vi "Scan Callers.vi"(8 "error in (no error)":errorcluster, 11 "WorkSpace / Repo path":path) -> (0 "error out":errorcluster)   [LabVIEW 2019, in "Hawkeye.lvlib"]
uses:
  Hawkeye.lvlib
panel:
  out "Dependency Chain [] 2":string[](array[string])
  in  "WorkSpace / Repo path 2":path
  out "Array 2":string[](array[string])
  out "Array 3":string[][](array[string])
  in  "Scan":bool
  in  "Status":string
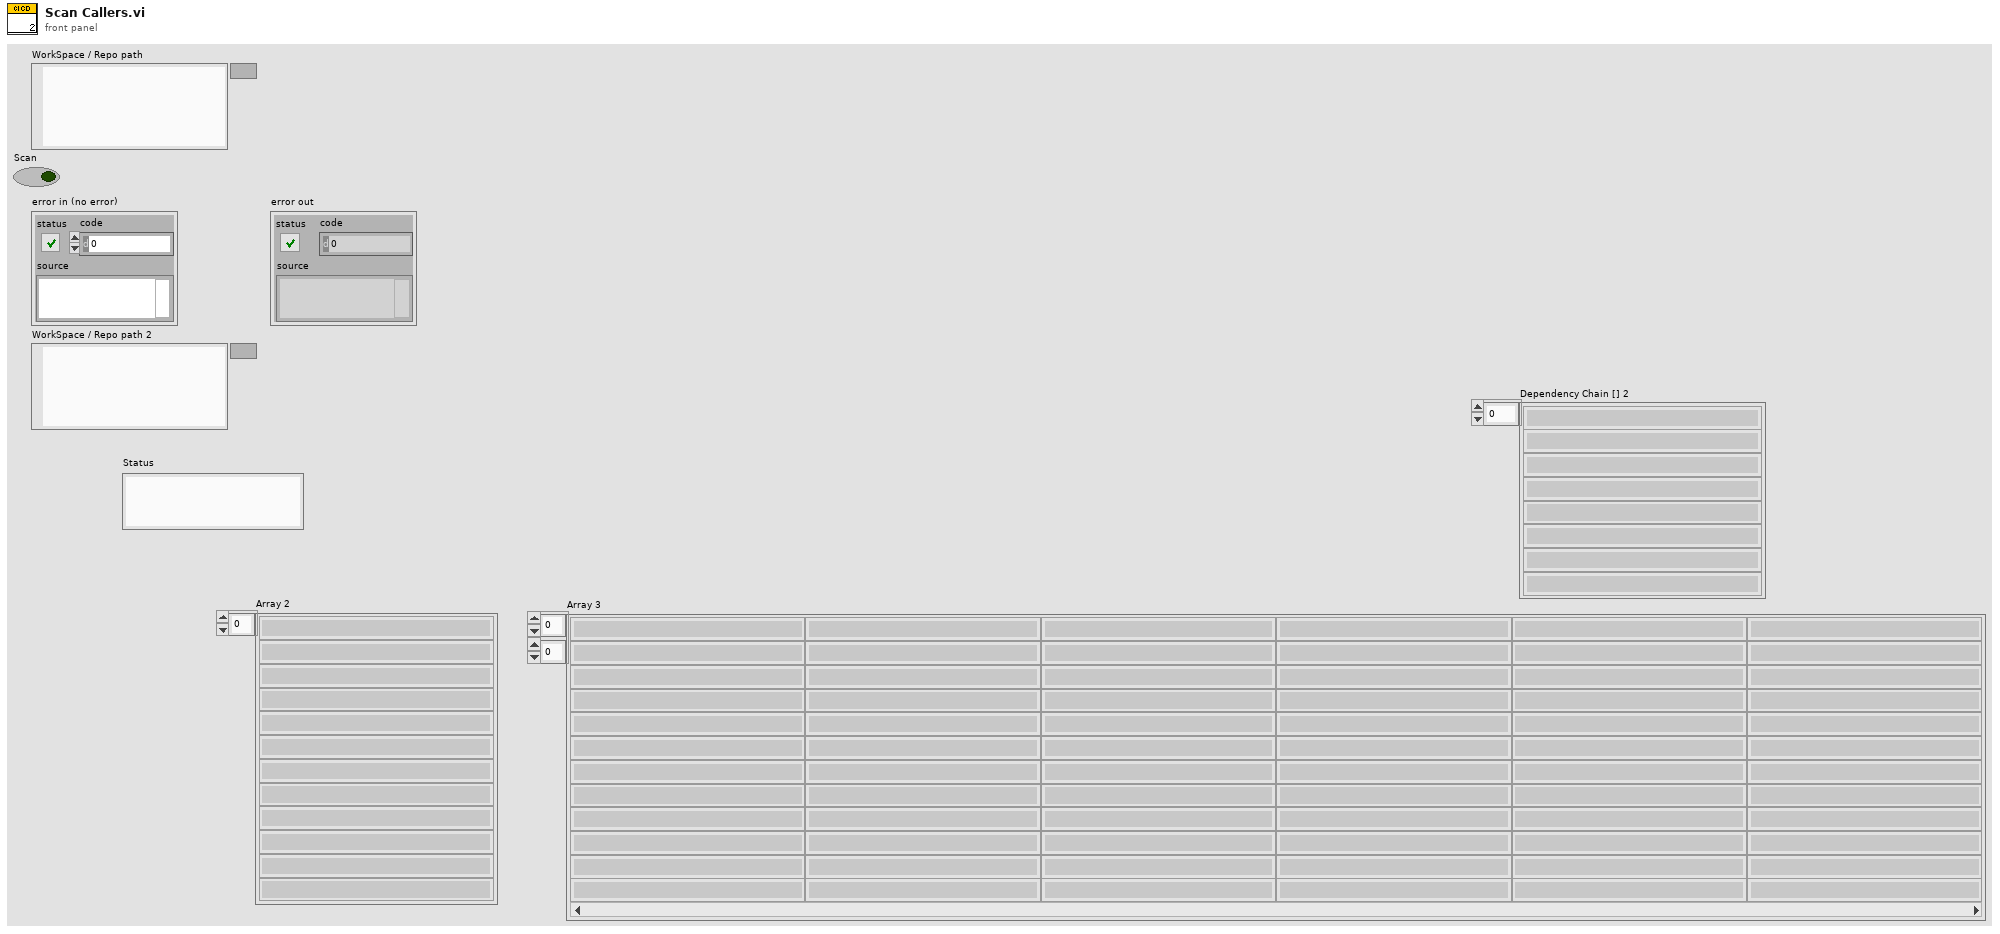
[diagram p1: front panel]
types:
  T1 = cluster{"VI Path":path, "Callees":set{string}, "LVLib/LVClass Name":string}[]
  T2 = enum16{"open", "replace", "create", "open or create", "replace or create", "replace or create with confirmation"}
  T3 = cluster{"VI Path":path, "Callees":set{string}, "LVLib/LVClass Name":string}
  T4 = typedef "NI_FileType.lvlib/LVFileType.ctl" = enum32{"Invalid file", "Unknown type", "Instrument", "Control", "Polymorphic VI", "Project", "Library", "LVClass", "XControl", "XNode", "Shared library", ".NET assembly", "ActiveX interface", "CIN", "Run-time menu", "Palette menu", "Help file", "LLB", "XNode Edit Dependency", "Class Private Data Control", "Statechart", "MathScript .m file", "Ladder Diagram", "LVLibp", "XNode Build Dependency"}
  T5 = cluster{"path":path, "delimited name":string, "type":T4, "iState":u32, "iStyle":u16, "wStyle":u16, "buttons":u16, "viflags":u32, "viflags2":u32, "links":u32[]}[]
  T6 = cluster{"path":path, "delimited name":string, "type":T4, "iState":u32, "iStyle":u16, "wStyle":u16, "buttons":u16, "viflags":u32, "viflags2":u32, "links":u32[]}
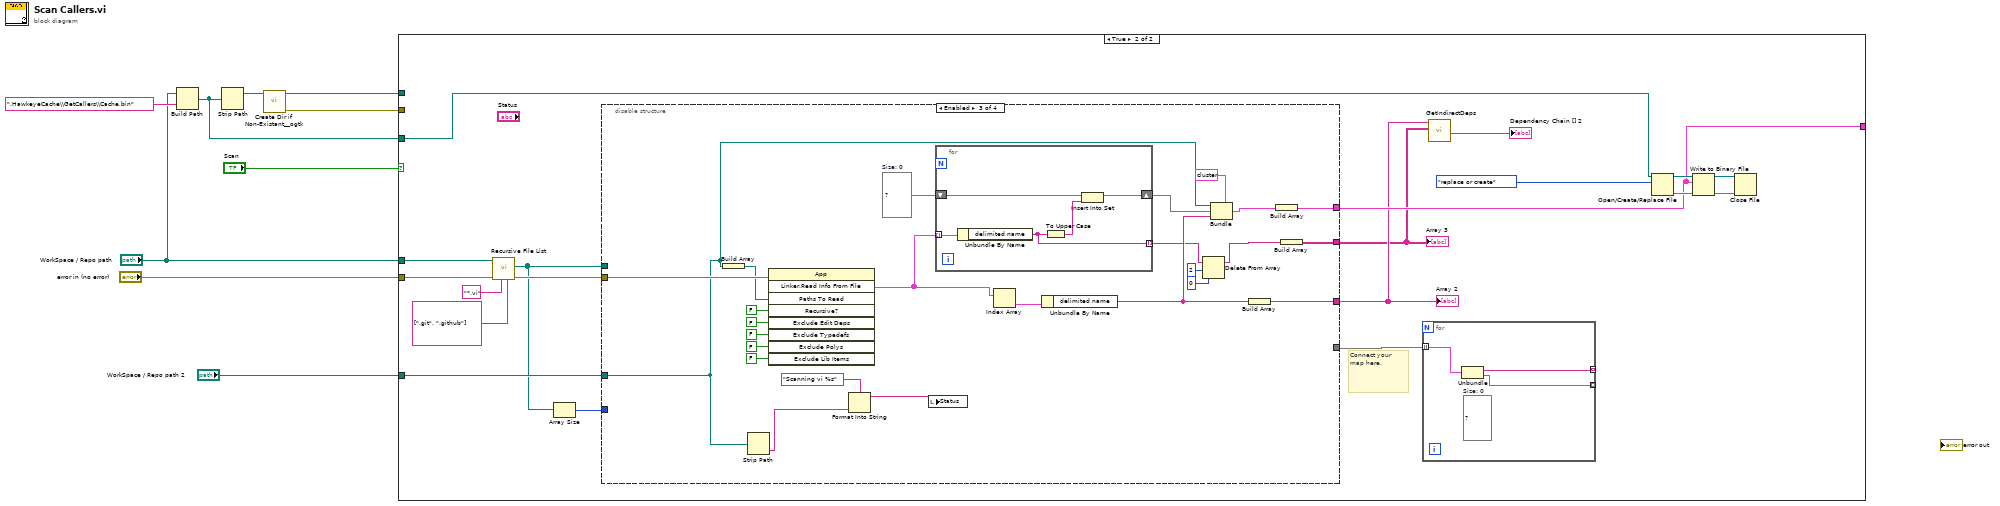
[diagram p0: block diagram]
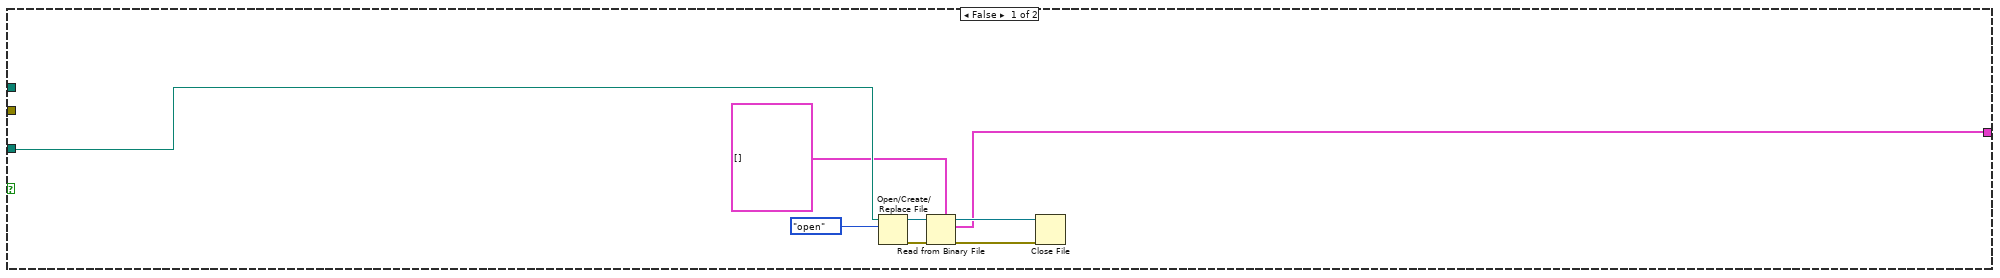
[diagram p2: hidden frame]
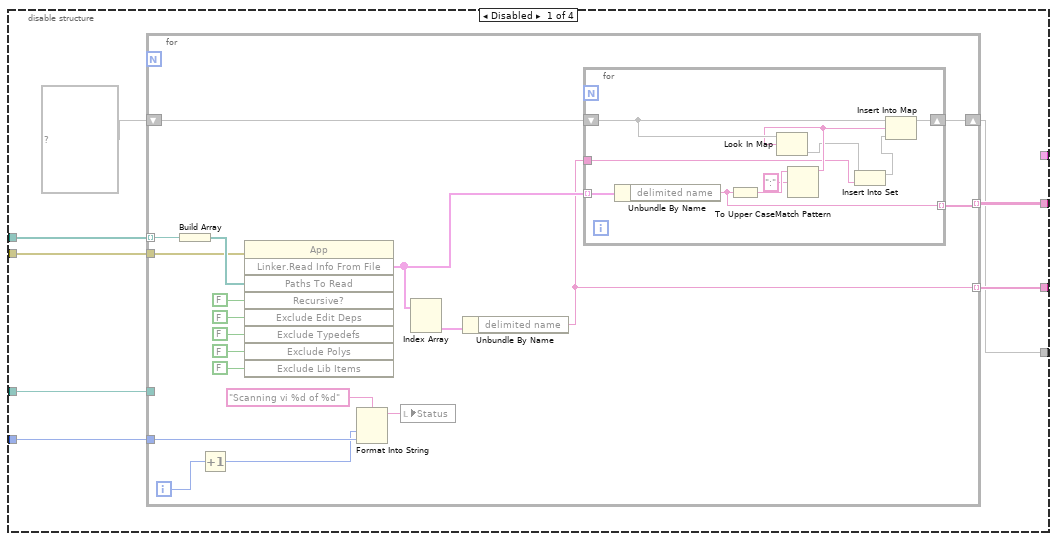
[diagram p3: hidden frame]
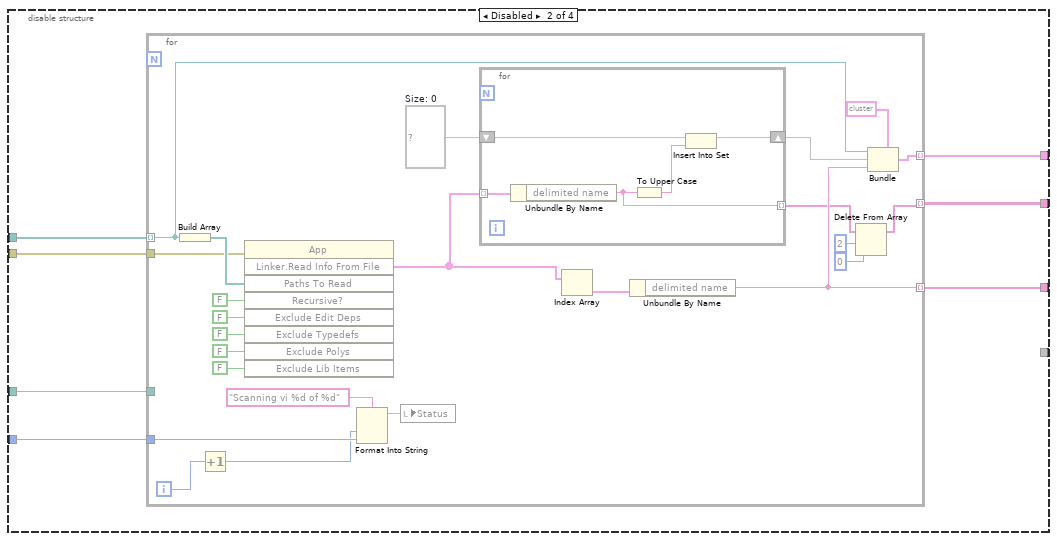
[diagram p4: hidden frame]
diagram:
  n1 = Build Path(base path="WorkSpace / Repo path", name or relative path=".HawkeyeCache\\GetCallers\\Cache.bin") -> (appended path=w2:path)
  n2 = Strip Path(path=w2) -> (stripped path=w5:path)  [unwired: 1 out]
  n3 = call <userlib>:"Create Dir if Non-Existant__ogtk.vi"("Directory Path"=w5) -> ("error out"=w4:errorcluster, "dup Directory Path"=w3:path)  [unwired: 8 in, 1 out]
  n4 = case shown="True" "Scan" {
    tunnel: "WorkSpace / Repo path" -> [_ w36]
    tunnel: "error in (no error)" -> [_ w35]
    tunnel: [w12 w26] -> _
    tunnel: w2 -> [w11 w25]
    tunnel: w4 -> [_ _]
    tunnel: w3 -> [_ _]
    tunnel: "WorkSpace / Repo path 2" -> [_ w23]
    frame False {
      n5 = Open/Create/Replace File(file path (use dialog)=w11, operation (0:open)=T2."open") -> (refnum out=w17:refnum<file>, error out=w13:errorcluster)  [unwired: 4 in, 1 out]
      n6 = Read from Binary File(5:T1 [] ("output cluster"), 8:w13, 11:w17) -> (0:w15:errorcluster, 2:w12:T1, 3:w16:refnum<file>)  [unwired: 3 in, 1 out]
      n7 = Close File(refnum=w16, error in=w15) -> ()  [unwired: 2 out]
    }
    frame True {
      # "Connect your map here."
      n8 = call <vilib>:"Recursive File List.vi"("Folders to Exclude"=string[] [".git", ".github"], "pattern"="*.vi", "error in (no error)"=w35, "Folder Path"=w36) -> ("error out"=w24:errorcluster, "All Files in Dir"=w22:path[])  [unwired: 3 in, 3 out]
      n9 = Array Size(array=w22) -> (size(s)=w32:i32)
      n10 = disable-structure shown="Enabled" {
        disable-tunnel: w32 -> [w47 w83 _ _]
        disable-tunnel: [_ w82 w115 _] -> w26
        disable-tunnel: [w46 w81 w114 _] -> w19
        disable-tunnel: w24 -> [w45 w80 w135 _]
        disable-tunnel: [w44 w79 w113 _] -> w20
        disable-tunnel: w23 -> [w43 w78 w117 _]
        disable-tunnel: w22 -> [w42 w77 _ _]
        disable-tunnel: [w40 _ _ _] -> w21
        frame Disabled {
          n11 = for {
            tunnel: w47 -> [w63]
            tunnel: [w55] -> w46 mode=indexing
            tunnel: w45 -> [w54]
            tunnel: [w49] -> w44 mode=indexing
            tunnel: w43 -> [_]
            tunnel: w42 -> [w51] mode=indexing
            shift-right: [w48] -> w40
            shift-left: map{string, set{string}} {} ("map in") -> [w50]
            i -> [w64]
            n12 = Build Array(w51) -> (w65:path[])
            n13 = Increment(x=w64) -> (x+1=w60:i32)
            n14 = invoke class="App" method="Linker.Read Info From File"(error in=w54, "Paths To Read"=w65, "Recursive?"=FALSE, "Exclude Edit Deps"=FALSE ("Exclude Edit Time Dependencies"), "Exclude Typedefs"=FALSE, "Exclude Polys"=FALSE ("Exclude Poly VIs"), "Exclude Lib Items"=FALSE ("Exclude Unused Library Items")) -> ("Linker.Read Info From File"=w53:T5)  [unwired: 2 in, 8 out]
            n15 = Format Into String(format string="Scanning vi %d of %d", w60, w63) -> (resulting string=w61:string)  [unwired: 2 in, 1 out]
            n16 = local write "Status"(w61) -> ()
            n17 = Index Array(array=w53) -> (element #2=w52:T6)  [unwired: 2 in, 1 out]
            n18 = Unbundle By Name(w52) -> ("delimited name"=w49:string)
            n19 = for {
              shift-right: [w73] -> w48
              shift-left: w50 -> [w74]
              tunnel: w53 -> [w76] mode=indexing
              tunnel: [w75] -> w55 mode=indexing
              tunnel: w49 -> [w68]
              n20 = Unbundle By Name(w76) -> ("delimited name"=w75:string)
              n21 = To Upper Case(1:w75) -> (0:w72:string)
              n22 = Match Pattern(string=w72, regular expression=":") -> (before substring=w70:string)  [unwired: 1 in, 3 out]
              n23 = Look In Map(map=w74, key=w70) -> (value=w69:set{string})  [unwired: 1 in, 1 out]
              n24 = Insert Into Set(10:w68, 11:w69) -> (3:w67:set{string})  [unwired: 1 out]
              n25 = Insert Into Map(map in=w74, key=w70, value=w67) -> (map out=w73:map{string, set{string}})  [unwired: 2 out]
            }
          }
        }
        frame Disabled {
          n26 = for {
            tunnel: w83 -> [w104]
            tunnel: [w98] -> w82 mode=indexing
            tunnel: [w85] -> w81 mode=indexing
            tunnel: w80 -> [w92]
            tunnel: [w89] -> w79 mode=indexing
            tunnel: w78 -> [_]
            tunnel: w77 -> [w88] mode=indexing
            i -> [w105]
            w101 = set{string} {}  # Size: 0
            n27 = Build Array(w88) -> (w106:path[])
            n28 = Increment(x=w105) -> (x+1=w97:i32)
            n29 = invoke class="App" method="Linker.Read Info From File"(error in=w92, "Paths To Read"=w106, "Recursive?"=FALSE, "Exclude Edit Deps"=FALSE ("Exclude Edit Time Dependencies"), "Exclude Typedefs"=FALSE, "Exclude Polys"=FALSE ("Exclude Poly VIs"), "Exclude Lib Items"=FALSE ("Exclude Unused Library Items")) -> ("Linker.Read Info From File"=w91:T5)  [unwired: 2 in, 8 out]
            n30 = Format Into String(format string="Scanning vi %d of %d", w97, w104) -> (resulting string=w102:string)  [unwired: 2 in, 1 out]
            n31 = local write "Status"(w102) -> ()
            n32 = for {
              shift-right: [w111] -> w100
              shift-left: w101 -> [w112]
              tunnel: w91 -> [w110] mode=indexing
              tunnel: [w108] -> w86 mode=indexing
              n33 = Unbundle By Name(w110) -> ("delimited name"=w108:string)
              n34 = To Upper Case(1:w108) -> (0:w109:string)
              n35 = Insert Into Set(10:w109, 11:w112) -> (3:w111:set{string})  [unwired: 1 out]
            }
            n36 = Index Array(array=w91) -> (element=w90:T6)  [unwired: 1 in]
            n37 = Unbundle By Name(w90) -> ("delimited name"=w89:string)
            n38 = Delete From Array(array=w86, length=2, index=0) -> (array with subset deleted=w85:string[])  [unwired: 1 out]
            n39 = Bundle(cluster=T3 {"VI Path"=path "", "Callees"={}, "LVLib/LVClass Name"=""} ("output cluster"), "VI Path"=w88, "Callees"=w100, "LVLib/LVClass Name"=w89) -> (w98:T3)
          }
        }
        frame Enabled {
          w129 = set{string} {}  # Size: 0
          n40 = Build Array(w117) -> (w132:path[])
          n41 = Strip Path(path=w117) -> (name=w116:string)  [unwired: 1 out]
          n42 = invoke class="App" method="Linker.Read Info From File"(error in=w135, "Paths To Read"=w132, "Recursive?"=FALSE, "Exclude Edit Deps"=FALSE ("Exclude Edit Time Dependencies"), "Exclude Typedefs"=FALSE, "Exclude Polys"=FALSE ("Exclude Poly VIs"), "Exclude Lib Items"=FALSE ("Exclude Unused Library Items")) -> ("Linker.Read Info From File"=w122:T5)  [unwired: 2 in, 8 out]
          n43 = Format Into String(format string="Scanning vi %s", w116) -> (resulting string=w130:string)  [unwired: 2 in, 1 out]
          n44 = local write "Status"(w130) -> ()
          n45 = for {
            shift-right: [w141] -> w128
            shift-left: w129 -> [w142]
            tunnel: w122 -> [w140] mode=indexing
            tunnel: [w138] -> w119 mode=indexing
            n46 = Unbundle By Name(w140) -> ("delimited name"=w138:string)
            n47 = To Upper Case(1:w138) -> (0:w139:string)
            n48 = Insert Into Set(10:w139, 11:w142) -> (3:w141:set{string})  [unwired: 1 out]
          }
          n49 = Index Array(array=w122) -> (element=w121:T6)  [unwired: 1 in]
          n50 = Unbundle By Name(w121) -> ("delimited name"=w134:string)
          n51 = Delete From Array(array=w119, length=2, index=0) -> (array with subset deleted=w136:string[])  [unwired: 1 out]
          n52 = Bundle(cluster=T3 {"VI Path"=path "", "Callees"={}, "LVLib/LVClass Name"=""} ("output cluster"), "VI Path"=w117, "Callees"=w128, "LVLib/LVClass Name"=w134) -> (w137:T3)
          n53 = Build Array(w134) -> (w113:string[])
          n54 = Build Array(w137) -> (w115:T1)
          n55 = Build Array(w136) -> (w114:string[][])
        }
        frame Disabled {
        }
      }
      "Array 3" <- w19
      "Array 2" <- w20
      n56 = for {
        tunnel: w21 -> [w39] mode=indexing
        tunnel: [w38] -> _ mode=indexing
        tunnel: [w37] -> _ mode=indexing
        (unwired) set{string} {}  # Size: 0
        n57 = Unbundle(w39) -> (w38:string, w37:set{string})
      }
      n58 = call "GetIndirectDeps.vi"("Descendents SubVIs Qualified Name"=w19, "LV Descendents Qualified Name"=w20) -> ("Dependency Chain [] 2"=→"Dependency Chain [] 2":string[])  [unwired: 8 in, 1 out]
      n59 = Open/Create/Replace File(file path (use dialog)=w25, operation (0:open)=T2."replace or create") -> (refnum out=w30:refnum<file>, error out=w27:errorcluster)  [unwired: 4 in, 1 out]
      n60 = Write to Binary File(file (use dialog)=w30, data=w26, error in=w27) -> (refnum out=w29:refnum<file>, error out=w28:errorcluster)  [unwired: 3 in, 1 out]
      n61 = Close File(refnum=w29, error in=w28) -> ()  [unwired: 2 out]
    }
  }
